vi "QueryServer_SetTestDataTypesResults.vi"(6 "error in (no error)":errorcluster, 8 "TestDataTypesParameters":T1, 9 "gRPCid":T3) -> (0 "error out":errorcluster, 3 "gRPCid out":T3)   [LabVIEW 2019, in "labview-grpc-query-server.lvlib"]
uses:
  labview-grpc-query-server.lvlib
  VIs/grpcId.ctl
  QueryServer_TestDataTypesParameters.ctl
  QueryServer_DataTypeTest.ctl
  d149c175-cf88-4dc1-b2b5-9725cea78de2.vi
  VIs/gprc-support.lvlib
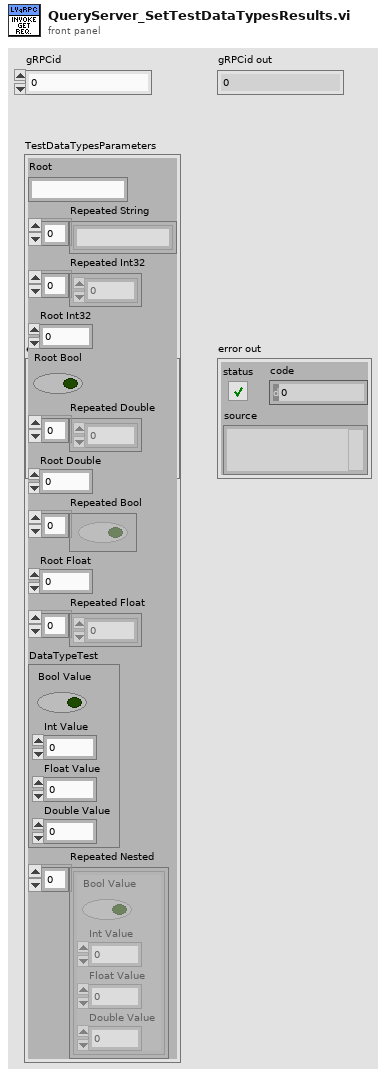
[diagram p1: front panel]
types:
  T1 = typedef "labview-grpc-query-server.lvlib/QueryServer_TestDataTypesParameters.ctl" = cluster{"Root":string, "Repeated String":string[], "Repeated Int32":i32[], "Root Int32":i32, "Root Bool":bool, "Repeated Double":dbl[], "Root Double":dbl, "Repeated Bool":bool[], "Root Float":sgl, "Repeated Float":sgl[], "DataTypeTest":T2, "Repeated Nested":T2[]}
  T2 = typedef "labview-grpc-query-server.lvlib/QueryServer_DataTypeTest.ctl" = cluster{"Bool Value":bool, "Int Value":i32, "Float Value":sgl, "Double Value":dbl}
  T3 = typedef "gprc-support.lvlib/grpcId.ctl" = u64
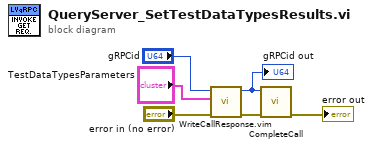
[diagram p0: block diagram]
diagram:
  n1 = call "WriteCallResponse.vim"("error in (no error)"="error in (no error)", "Response Data"="TestDataTypesParameters", "gRPCid in"="gRPCid") -> ("error out"=w5:errorcluster, "gRPCid"=w3:T3)  [unwired: 7 in]
  "gRPCid out" <- w3
  n2 = call "CompleteCall.vi"("gRPCid"=w3, "error in (no error)"=w5) -> ("error out"=→"error out":errorcluster)  [unwired: 8 in]
